vi "scan_mem_helper.vi"(8 "error in (no error)":errorcluster, 9 "scan_desc":T2, 10 "chav":T1[](array[typedef]), 11 "DAQ ID":string="usbbase") -> (0 "error out":errorcluster, 1 "scan_desc out":T2, 2 "chav out":T1[](array[typedef]), 3 "buffer out":sgl[][](array[numeric]))   [LabVIEW 2021, in "libad4.lvlib"]
doc: "Helper function to perform in-memory DAQ scan."
uses:
  <userlib>/libad4/libad4.lvlib
  <userlib>/libad4/controls/ad scan cha desc.ctl
  <userlib>/libad4/controls/ad scan desc.ctl
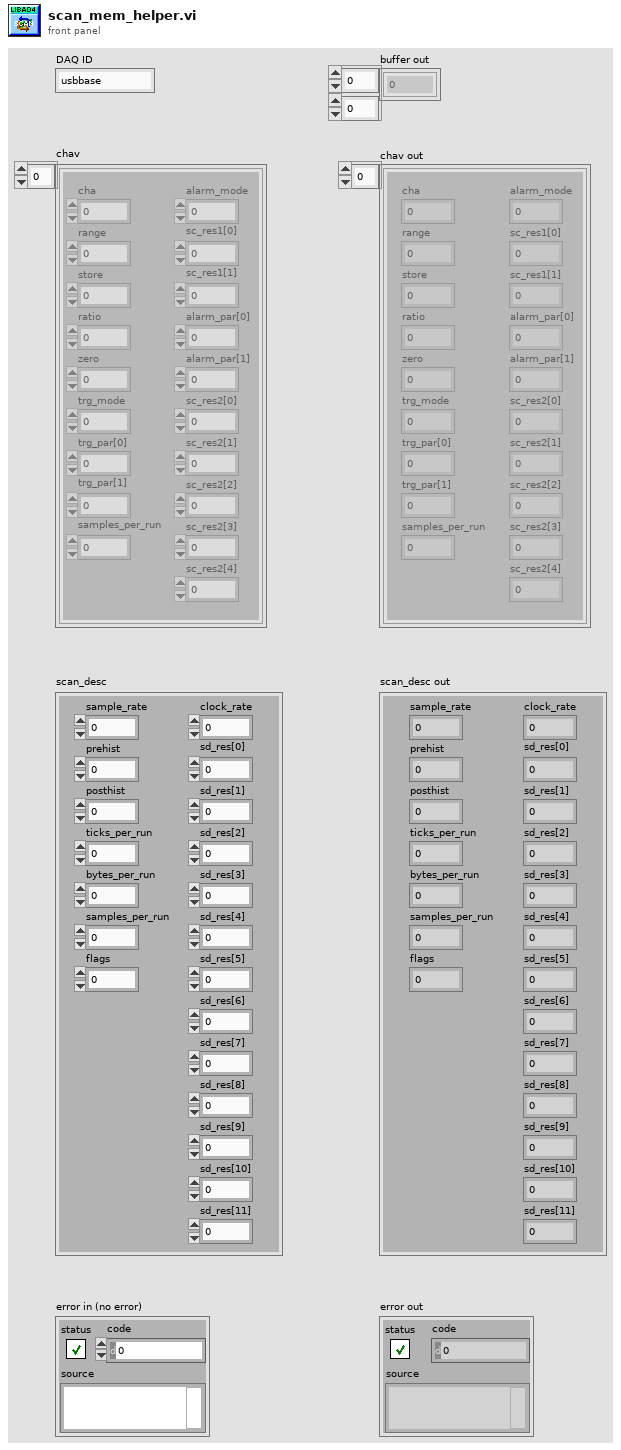
[diagram p1: front panel]
types:
  T1 = typedef "libad4.lvlib/ad scan cha desc.ctl" = cluster{"cha":i32, "range":i32, "store":i32, "ratio":i32, "zero":u32, "trg_mode":u8, "alarm_mode":u8, "sc_res1[0]":u8, "sc_res1[1]":u8, "trg_par[0]":u32, "trg_par[1]":u32, "samples_per_run":i32, "alarm_par[0]":u32, "alarm_par[1]":u32, "sc_res2[0]":u32, "sc_res2[1]":u32, "sc_res2[2]":u32, "sc_res2[3]":u32, "sc_res2[4]":u32}
  T2 = typedef "libad4.lvlib/ad scan desc.ctl" = cluster{"sample_rate":dbl, "clock_rate":dbl, "prehist":u64, "posthist":u64, "ticks_per_run":u32, "bytes_per_run":u32, "samples_per_run":u32, "flags":u32, "sd_res[0]":u32, "sd_res[1]":u32, "sd_res[2]":u32, "sd_res[3]":u32, "sd_res[4]":u32, "sd_res[5]":u32, "sd_res[6]":u32, "sd_res[7]":u32, "sd_res[8]":u32, "sd_res[9]":u32, "sd_res[10]":u32, "sd_res[11]":u32}
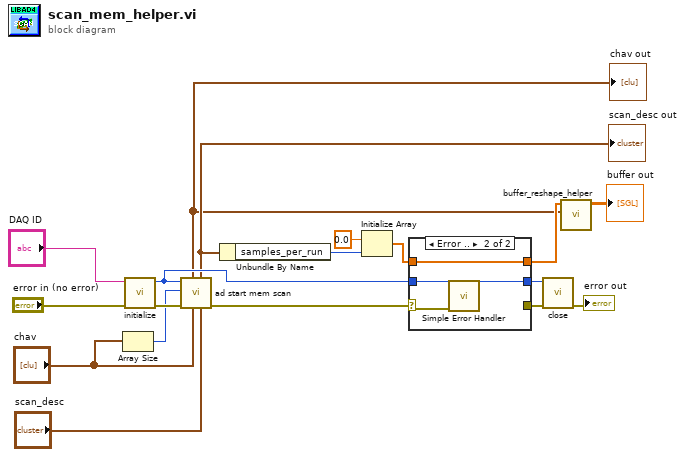
[diagram p0: block diagram]
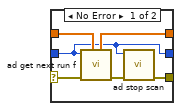
[diagram p2: hidden frame]
diagram:
  n1 = Array Size(array="chav") -> (size(s)=w8:i32)
  n2 = call <userlib>:"initialize.vi"("error in (no error)"="error in (no error)", "name"="DAQ ID") -> ("error out"=w14:errorcluster, "function return"=w17:i32)  [unwired: 8 in]
  n3 = call <userlib>:"ad start mem scan.vi"("sd"="scan_desc", "chav"="chav", "error in (no error)"=w14, "chac"=w8, "adh"=w17) -> ("error out"=w12:errorcluster, "sd out"=w4:T2, "chav out"=w2:T1[])  [unwired: 3 in, 1 out]
  "scan_desc out" <- w4
  "chav out" <- w2
  n4 = Unbundle By Name(w4) -> ("samples_per_run"=w7:u32)
  n5 = Initialize Array(sgl 0.0 ("element"), w7) -> (w5:sgl[])
  n6 = case shown="Error .." w12 {
    selector: w12 -> [w24 w25]
    tunnel: w17 -> [w19 w27]
    tunnel: [w22 _] -> w15
    tunnel: w5 -> [w21 w26]
    tunnel: [w20 w26] -> w3
    tunnel: [w19 w27] -> w18
    frame No Error {
      n7 = call <userlib>:"ad get next run f.vi"("buffer"=w21, "error in (no error)"=w24, "adh"=w19) -> ("error out"=w23:errorcluster, "buffer out"=w20:sgl[])  [unwired: 4 in, 3 out]
      n8 = call <userlib>:"ad stop scan.vi"("error in (no error)"=w23, "adh"=w19) -> ("error out"=w22:errorcluster)  [unwired: 7 in, 2 out]
    }
    frame Error {
      n9 = call <vilib>:"Simple Error Handler.vi"("error in (no error)"=w25) -> ()  [unwired: 4 in, 5 out]
    }
  }
  n10 = call <userlib>:"close.vi"("error in (no error)"=w15, "adh"=w18) -> ("error out"=→"error out":errorcluster)  [unwired: 8 in, 1 out]
  n11 = call <userlib>:"buffer_reshape_helper.vi"("chav in"=w2, "p in"=w3) -> ("buffer out"=→"buffer out":sgl[][])  [unwired: 9 in]
